vi "IND560 Standalone Checker.vi"(0 "VISA resource name":refnum<visa-resource-name>="IND560") -> (4 "Displayed Gross Wt.":dbl, 6 "Displayed Net Wt.":dbl)   [LabVIEW 2016]
panel:
  out "IND560 Scale Data Runtime":string[][](array[string])
  out "appended array":string[][](array[string])
  in  "stop 2":bool
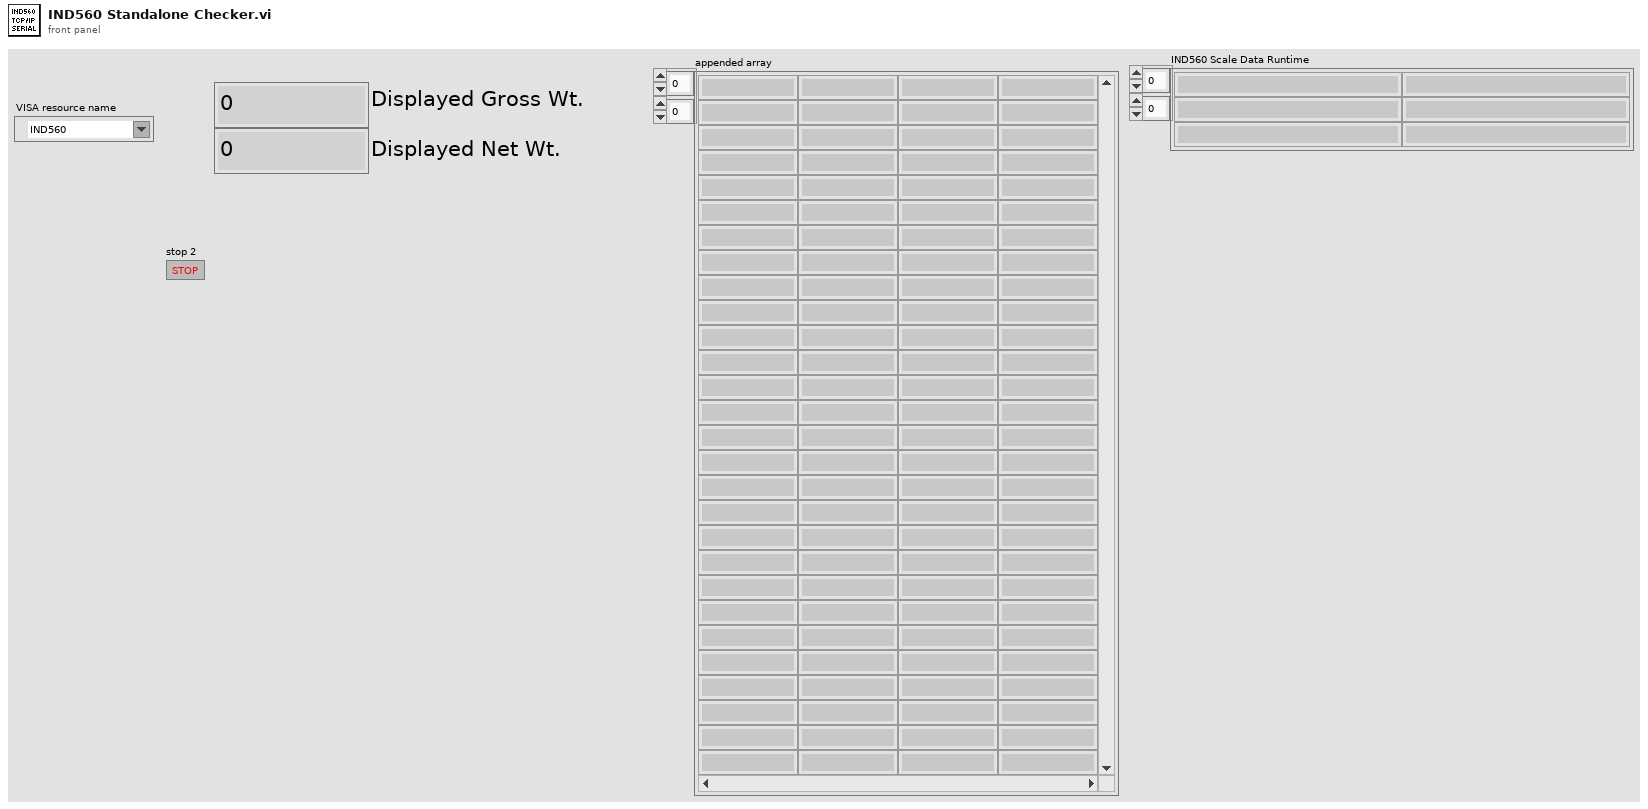
[diagram p1: front panel]
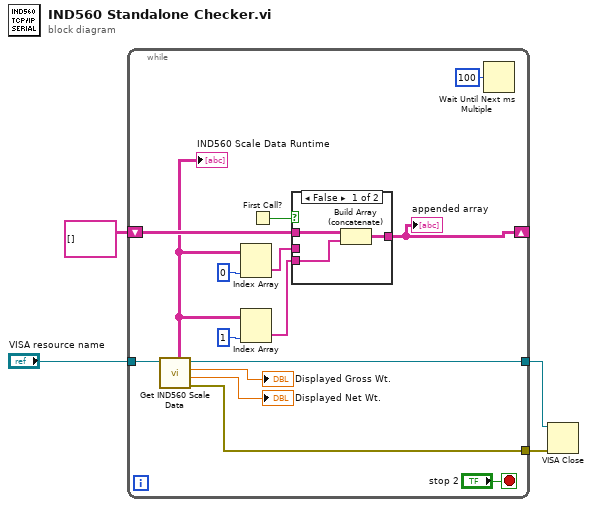
[diagram p0: block diagram]
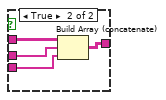
[diagram p2: hidden frame]
diagram:
  n1 = while {
    tunnel: "VISA resource name" -> [w18]
    tunnel: [w16] -> w1
    shift-right: [w12] -> _
    shift-left: string[][] [] -> [w13]
    tunnel: [w5] -> w2
    stop <- "stop 2" stop-if-true
    n2 = call "Get IND560 Scale Data.vi"("VISA Refnum in"=w18) -> ("error out"=w16:errorcluster, "Displayed Net Wt."=→"Displayed Net Wt.":dbl, "Displayed Gross Wt."=→"Displayed Gross Wt.":dbl, "VISA Refnum out"=w5:refnum<visa-resource-name>, "IND560 Scale Data"=w11:string[][])  [unwired: 6 in]
    "IND560 Scale Data Runtime" <- w11
    n3 = Index Array(array=w11, index (col)=0 ("index (row)")) -> (element=w8:string[])  [unwired: 1 in]
    n4 = Index Array(array=w11, index (col)=1 ("disabled index (col)")) -> (element=w7:string[])  [unwired: 1 in]
    n5 = First Call?() -> (First Call?: T/F=w10:bool)
    n6 = case shown="False" w10 {
      tunnel: w13 -> [w22 w26]
      tunnel: [w21 w25] -> w12
      tunnel: w8 -> [_ w24]
      tunnel: w7 -> [w20 w23]
      frame False {
        n7 = Build Array (concatenate)(w22, w20) -> (w21:string[][])
      }
      frame True {
        n8 = Build Array (concatenate)(w26, w24, w23) -> (w25:string[][])
      }
    }
    "appended array" <- w12
    n9 = Wait Until Next ms Multiple(millisecond multiple=u32 100) -> ()  [unwired: 1 out]
  }
  n10 = VISA Close(VISA resource name=w2, error in (no error)=w1) -> ()  [unwired: 1 out]
